vi "Swerve_Module_Setup.vi"   [LabVIEW 2020]
uses:
  Robot Global Data.vi
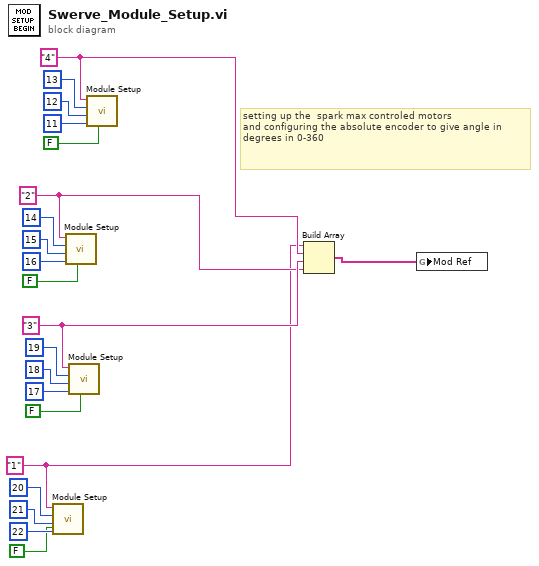
[diagram p0: block diagram]
diagram:
  w5 = "1" ("string")
  w8 = "3" ("string")
  w7 = "2" ("string")
  w9 = "4" ("string")
  # "setting up the  spark max controled motors\nand configuring the absolute encoder to give angle in \ndegrees in 0-360"
  n1 = call "Module Setup.vi"("Invert"=FALSE, "Vel ID 2"=u8 22, "Vel ID"=u8 21 ("Device Number"), "Rot ID"=u8 20 ("Device Number"), "Mod Des"=w5) -> ()  [unwired: 7 in]
  n2 = call "Module Setup.vi"("Invert"=FALSE, "Vel ID 2"=u8 16, "Vel ID"=u8 15 ("Device Number"), "Rot ID"=u8 14 ("Device Number"), "Mod Des"=w7) -> ()  [unwired: 7 in]
  n3 = call "Module Setup.vi"("Invert"=FALSE, "Vel ID 2"=u8 17, "Vel ID"=u8 18 ("Device Number"), "Rot ID"=u8 19 ("Device Number"), "Mod Des"=w8) -> ()  [unwired: 7 in]
  n4 = call "Module Setup.vi"("Invert"=FALSE, "Vel ID 2"=u8 11, "Vel ID"=u8 12 ("Device Number"), "Rot ID"=u8 13 ("Device Number"), "Mod Des"=w9) -> ()  [unwired: 7 in]
  n5 = Build Array(w5, w9, w8, w7) -> (w6:string[])
  n6 = global write "Robot Global Data.vi" "Mod Ref"(w6) -> ()
